vi "Logger Report Errors.vi"(11 "error in (no error)":errorcluster) -> (15 "error out":errorcluster)   [LabVIEW 2018]
uses:
  Logger Global.vi
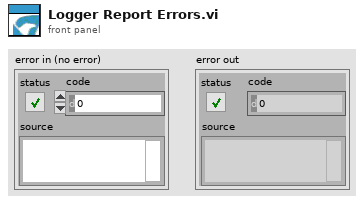
[diagram p1: front panel]
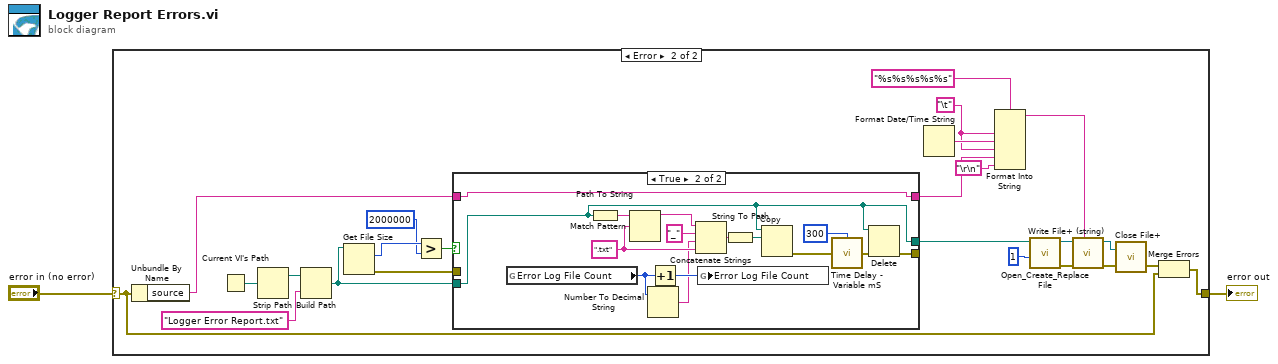
[diagram p0: block diagram]
diagram:
  n1 = case shown="Error" "error in (no error)" {
    selector: "error in (no error)" -> [w3 w16]
    tunnel: [w3 w17] -> w1
    frame No Error {
    }
    frame Error {
      w19 = "\t"
      n2 = Unbundle By Name(w16) -> ("source"=w12:string)
      n3 = Current VI's Path() -> (path=w14:path)
      n4 = Strip Path(path=w14) -> (stripped path=w13:path)  [unwired: 1 out]
      n5 = Build Path(base path=w13, name or relative path="Logger Error Report.txt") -> (appended path=w5:path)
      n6 = Get File Size(file=w5) -> (size (in bytes)=w9:i64, 0:w4:errorcluster)  [unwired: 1 in, 1 out]
      n7 = Greater?(x=w9, y=i64 2000000) -> (0:w7:bool)
      n8 = case shown="True" w7 {
        tunnel: w12 -> [w29 w44]
        tunnel: [w29 w44] -> w11
        tunnel: w5 -> [w28 w33]
        tunnel: [_ w34] -> _
        tunnel: [w28 w33] -> w6
        tunnel: w4 -> [_ _]
        frame False {
        }
        frame True {
          w32 = ".txt" ("regular expression")
          n9 = global read "Logger Global.vi" "Error Log File Count"() -> (w38:u16)
          n10 = Path To String(path=w33) -> (string=w39:string)
          n11 = Match Pattern(string=w39, regular expression=w32) -> (before substring=w37:string)  [unwired: 1 in, 3 out]
          n12 = Number To Decimal String(number=w38) -> (decimal integer string=w31:string)  [unwired: 1 in]
          n13 = Increment(x=w38) -> (x+1=w43:u16)
          n14 = Concatenate Strings(w37, "_" ("string"), w31, w32) -> (w36:string)
          n15 = global write "Logger Global.vi" "Error Log File Count"(w43) -> ()
          n16 = String To Path(string=w36) -> (path=w35:path)
          n17 = Copy(10:w35, 11:w33) -> (0:w41:errorcluster)  [unwired: 3 in, 2 out]
          n18 = call "Time Delay - Variable mS.vi"("milliseconds to wait"=u32 300, "error in (no error)"=w41) -> ("error out"=w40:errorcluster)  [unwired: 2 in]
          n19 = Delete(path (use dialog)=w33, error in=w40) -> (error out=w34:errorcluster)  [unwired: 3 in, 2 out]
        }
      }
      n20 = Format Date/Time String() -> (date/time string=w20:string)  [unwired: 3 in]
      n21 = Format Into String(format string="%s%s%s%s%s", w19, w20, w19, w11, "\r\n") -> (resulting string=w18:string)  [unwired: 2 in, 1 out]
      n22 = call <vilib>:"Open_Create_Replace File.vi"("function (open:0)"=1, "file path"=w6) -> ("error out"=w24:errorcluster, "refnum"=w26:refnum<file>)  [unwired: 6 in, 2 out]
      n23 = call <vilib>:"Write File+ (string).vi"("string"=w18, "error in (no error)"=w24, "refnum"=w26) -> ("error out"=w23:errorcluster, "dup refnum"=w27:refnum<file>)  [unwired: 4 in, 1 out]
      n24 = call <vilib>:"Close File+.vi"("error in (no error)"=w23, "refnum"=w27) -> ("error out"=w22:errorcluster)  [unwired: 3 in, 2 out]
      n25 = Merge Errors(w22, w16) -> (w17:errorcluster)
    }
  }
  "error out" <- w1
